vi "New Algo integrated.vi"(0 "Result data in":T6={"Measurement Names Array"=[], "Pass-Fail Array"=[], "Measurement Values Array "=[], "Roi for overlay (Arrows) Array"=[], "Algo Type Array"=[], "Image Array"=[], "Clamp operations"=enum."Average Clamp", "  Search Direction "=[], "Images_Array_in"=[], "ResultPF"=FALSE, "Total Cluster Values"={"Total Fail"=0, "Total Pass"=0, "Total Count"=0}, "Reel Counter Cluster"={"Reel Fail"=0, "Reel Pass"=0, "Reel Count"=0}, "Tolerance  Array"=[], "Array of Cam Spec Control Bool"=[], "Control Pass Fail Array"=[], "Specification Pass Fail Array"=[], "Overlay Arrow Lines"=[], "Camera ID"=[], "Trigger count"=0, "Specification fail?"=FALSE}, 1 "Measurements":T3, 2 "Coordinate Other Cluster":T1, 4 "Calibrated Image":T5[](array[typedef]), 5 "Co Ordinate System":T2(array[cluster]), 7 "error in":errorcluster) -> (21 "Spec Values":T4(array[cluster]), 25 "Result data out":T6={"Measurement Names Array"=[], "Pass-Fail Array"=[], "Measurement Values Array "=[], "Roi for overlay (Arrows) Array"=[], "Algo Type Array"=[], "Image Array"=[], "Clamp operations"=enum."Average Clamp", "  Search Direction "=[], "Images_Array_in"=[], "ResultPF"=FALSE, "Total Cluster Values"={"Total Fail"=0, "Total Pass"=0, "Total Count"=0}, "Reel Counter Cluster"={"Reel Fail"=0, "Reel Pass"=0, "Reel Count"=0}, "Tolerance  Array"=[], "Array of Cam Spec Control Bool"=[], "Control Pass Fail Array"=[], "Specification Pass Fail Array"=[], "Overlay Arrow Lines"=[], "Camera ID"=[], "Trigger count"=0, "Specification fail?"=FALSE}, 27 "error Out":errorcluster)   [LabVIEW 2019, in "Algorithm.lvclass"]
uses:
  FrameworkOverrides/Algorithm.lvclass
  <vilib>/vision/NI_Vision_Development_Module.lvlib
  <vilib>/vision/Image Controls.llb/IMAQ Image.ctl
  Controls/Result Cluster.ctl
  Controls/Measurements JSON Read.ctl
panel:
  out "Numeric":i32
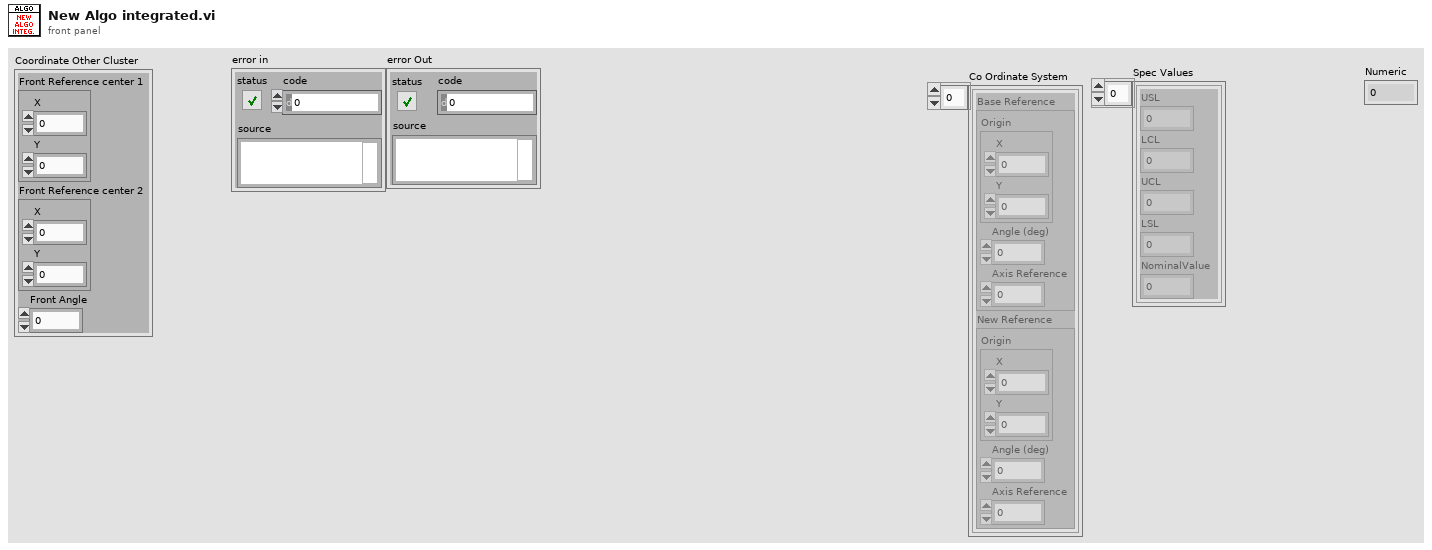
[diagram p1: front panel]
types:
  T1 = cluster{"Front Reference center 1":cluster{"X":sgl, "Y":sgl}, "Front Reference center 2":cluster{"X":sgl, "Y":sgl}, "Front Angle":dbl}
  T2 = cluster{"Base Reference":cluster{"Origin":cluster{"X":sgl, "Y":sgl}, "Angle (deg)":sgl, "Axis Reference":u32}, "New Reference":cluster{"Origin":cluster{"X":sgl, "Y":sgl}, "Angle (deg)":sgl, "Axis Reference":u32}}[]
  T3 = typedef "Algorithm.lvclass/Measurements JSON Read.ctl" = cluster{"RackID":i32, "ImageID":i32, "CameraID":i32, "MeasurementId":i32, "Name":string, "AlgoName":string, "Type":string, "MeasurementEnable":bool, "AlgorithmSequence":cluster{"RefernceEdge":cluster{"Enable":bool, "Method":string, "RefROI":cluster{"Left":i32, "Top":i32, "Right":i32, "Bottom":i32, "Rotation":dbl}, "EdgeOptions":cluster{"EdgePoarity":i32, "KernelSize":i32, "Width":i32, "MinimumEdgeStrength":i32, "InterpolationType":i32, "DataProcessingMethod":i32}, "LineOptions":cluster{"NumberofLines":i32, "Type":i32, "MinScore":i32, "MaxScore":i32, "Orientation":i32, "AngleRange":i32, "AngleTolerance":i32, "StepSize":i32, "MinSNR":i32, "MinPoints":i32, "HoughIterations":i32}, "SearchDirection":i32}, "Measurement":cluster{"ROI1":cluster{"Enable":bool, "ROI":cluster{"Left":i32, "Top":i32, "Right":i32, "Bottom":i32, "Rotation":dbl}, "EdgeOptions":cluster{"EdgePoarity":i32, "KernelSize":i32, "Width":i32, "MinimumEdgeStrength":i32, "InterpolationType":i32, "DataProcessingMethod":i32}, "LineOptions":cluster{"NumberofLines":i32, "Type":i32, "MinScore":i32, "MaxScore":i32, "Orientation":i32, "AngleRange":i32, "AngleTolerance":i32, "StepSize":i32, "MinSNR":i32, "MinPoints":i32, "HoughIterations":i32}, "Process":i32, "StepSize":i32, "SearchDirection":i32, "CircleEdgeOptions":cluster{"SearchDirection":i32, "EdgeOptions":cluster{"EdgePoarity":i32, "KernelSize":i32, "Width":i32, "MinimumEdgeStrength":i32, "InterpolationType":i32, "DataProcessingMethod":i32}}, "CircleFitOptions":cluster{"Process":i32, "StepSize":i32, "MAxPixelRadius":dbl}, "CircleSearchDirection":i32, "CurveParameters":cluster{"ExtractionMode":i32, "EdgeThreshold":i32, "EdgeFilterSize":i32, "MinLength":i32, "RowSearchStepSize":i32, "ColSearchStepSize":i32, "MaxEndpointGap":i32, "Closed":bool, "Subpixel":bool}, "MinimumMatchScore":i32, "CircleDescriptor":cluster{"MinRadius":i32, "MaxRadius":i32}, "EllipseDescriptor":cluster{"MinMajorRadius":i32, "MaxMajorRadius":i32, "MinMinorRadius":i32, "MaxMinorRadius":i32}}, "ROI2":cluster{"Enable":bool, "ROI":cluster{"Left":i32, "Top":i32, "Right":i32, "Bottom":i32, "Rotation":dbl}, "EdgeOptions":cluster{"EdgePoarity":i32, "KernelSize":i32, "Width":i32, "MinimumEdgeStrength":i32, "InterpolationType":i32, "DataProcessingMethod":i32}, "LineOptions":cluster{"NumberofLines":i32, "Type":i32, "MinScore":i32, "MaxScore":i32, "Orientation":i32, "AngleRange":i32, "AngleTolerance":i32, "StepSize":i32, "MinSNR":i32, "MinPoints":i32, "HoughIterations":i32}, "Process":i32, "StepSize":i32, "SearchDirection":i32, "CircleEdgeOptions":cluster{"SearchDirection":i32, "EdgeOptions":cluster{"EdgePoarity":i32, "KernelSize":i32, "Width":i32, "MinimumEdgeStrength":i32, "InterpolationType":i32, "DataProcessingMethod":i32}}, "CircleFitOptions":cluster{"Process":i32, "StepSize":i32, "MAxPixelRadius":dbl}, "CircleSearchDirection":i32, "CurveParameters":cluster{"ExtractionMode":i32, "EdgeThreshold":i32, "EdgeFilterSize":i32, "MinLength":i32, "RowSearchStepSize":i32, "ColSearchStepSize":i32, "MaxEndpointGap":i32, "Closed":bool, "Subpixel":bool}, "MinimumMatchScore":i32, "CircleDescriptor":cluster{"MinRadius":i32, "MaxRadius":i32}, "EllipseDescriptor":cluster{"MinMajorRadius":i32, "MaxMajorRadius":i32, "MinMinorRadius":i32, "MaxMinorRadius":i32}}}}, "MathExpression":cluster{"Algorithm":string, "MathExpression":string, "ResultVariable":string}, "MathCorrectionParameters":cluster{"Radius":dbl, "CurlGap":dbl, "Thickness":dbl, "MeasurementIndices":i32[], "MathAlgoName":string, "MathAlgoFormula":string, "CorrectionForAngle":i32[], "NumericAray":i32[], "StringArray":string[]}, "ResultVariableCluster":cluster{"RVName":string, "RVSequence":string, "RVIndex":i32, "RVID":i32, "RVValue":dbl}, "CalibrationCoefficients":cluster{"A1":dbl, "A2":dbl, "A3":dbl}, "UserCalibCoefficients":cluster{"UserCorrectionLinearityCoeff":dbl, "UserCorrectionBiasCoeff":dbl}, "SpecValues":cluster{"LCL":dbl, "UCL":dbl, "LSL":dbl, "USL":dbl, "NominalValue":dbl}, "OverlayOptions":cluster{"OverlayEnable":bool, "OverlayText":string, "OverlayCoords":i32[], "OverlayAngle":i32, "OverlayTextSize":i32, "OverlayTextColor":string, "OverlayROI":bool, "OverlayRakeLine":bool, "OverlayPoints":bool}, "DatalogEnable":bool, "DisplayIcon":string}[]
  T4 = cluster{"USL":dbl, "LCL":dbl, "UCL":dbl, "LSL":dbl, "NominalValue":dbl}[]
  T5 = typedef "IMAQ Image.ctl" = refnum<image>
  T6 = typedef "Algorithm.lvclass/Result Cluster.ctl" = cluster{"Measurement Names Array":string[], "Pass-Fail Array":bool[], "Measurement Values Array ":dbl[], "Roi for overlay (Arrows) Array":cluster{"Points for Arrow Overlay[0]":cluster{"x":dbl, "y":dbl}, "Points for Arrow Overlay[1]":cluster{"x":dbl, "y":dbl}, "Points for Arrow Overlay[2]":cluster{"x":dbl, "y":dbl}, "Points for Arrow Overlay[3]":cluster{"x":dbl, "y":dbl}}[], "Algo Type Array":string[], "Image Array":string[], "Clamp operations":enum16{"Min Clamp", "Max Clamp", "Average Clamp"}, "  Search Direction ":enum16{"Left to Right", "Right to Left", "Top to Bottom", "Bottom to Top"}[], "Images_Array_in":T5[], "ResultPF":bool, "Total Cluster Values":cluster{"Total Fail":u64, "Total Pass":u64, "Total Count":u64}, "Reel Counter Cluster":cluster{"Reel Fail":u64, "Reel Pass":u64, "Reel Count":u64}, "Tolerance  Array":string[], "Array of Cam Spec Control Bool":cluster{"Specification Boolean":bool, "Control Boolean":bool, "Camera ID":i8}[], "Control Pass Fail Array":bool[], "Specification Pass Fail Array":bool[], "Overlay Arrow Lines":cluster{"First Overlay Line ":cluster{"Start Point":cluster{"X":sgl, "Y":sgl}, "Start Point":cluster{"X":sgl, "Y":sgl}}, "Second Overlay Line ":cluster{"Start Point":cluster{"X":sgl, "Y":sgl}, "Start Point":cluster{"X":sgl, "Y":sgl}}}[], "Camera ID":i8[], "Trigger count":i32, "Specification fail?":bool}
  T7 = typedef "ROI Descriptor" = cluster{"Global Rectangle":i32[], "Contours":cluster{"ID":enum32{"External", "Internal"}, "Type":u32, "Coordinates":i32[]}[]}
  T8 = cluster{"ROI Ref [ After Transformation]":T7, "Measurement ROI 1 [After Transformation]":T7, "Measurement ROI 2 [After Transformation]":T7}
  T9 = typedef "Edge Options.ctl" = cluster{"Edge Polarity":T10, "Kernel Size":u32, "Width":u32, "Minimum Edge Strength":sgl, "Interpolation Type":enum32{"Zero Order", "Bilinear", "Quadratic", "Cubic", "Bilinear Fixed"}, "Data Processing Method":enum32{"Average", "Median"}}
  T10 = typedef "Edge Polarity.ctl" = u32
  T11 = typedef "Straight Edge Options.ctl" = cluster{"Number of Lines":i32, "Type":T12, "Min. Score":dbl, "Max. Score":dbl, "Orientation":dbl, "Angle Range":dbl, "Angle Tolerance":dbl, "Step Size":u32, "Min. SNR (db)":dbl, "Min. Points (%)":dbl, "Hough Iterations":i32}
  T12 = typedef "Straight Edge Process.ctl" = enum32{"First Edge Rake", "Best Edge Rake", "Hough Edge Rake", "First Edge Projection", "Best Edge Projection"}
  T13 = cluster{"RackID":i32, "ImageID":i32, "CameraID":i32, "MeasurementID":i32, "Measurement Name":string, "Algo Name":string, "Algo Type":string, "Ref ROI Cluster":cluster{"ROI Ref":cluster{"Global Rectangle":i32[], "Contours":cluster{"ID":enum32{"External", "Internal"}, "Type":u32, "Coordinates":i32[]}[]}, "Edge Options ROI Ref":T9, "Line Options ROI Ref":T11, "Search Direction ROI Ref":u32, "RefROIEnable":bool}, "Measurement ROI 1 Cluster":cluster{"Meas ROI 1":T7, "Edge Options ROI 1":T9, "Line Options ROI 1":T11, "Scan/Search Direction ROI 1":u16, "Step Size ROI 1":u32, "Process ROI 1":enum16{"Get First Edge", "Get First + Last Edge", "Get All Edges", "Get Best Edge"}, "Circle Options ROI 1":cluster{"Search  Direction":u32, "Edge Options":T9, "Show Search Area":bool, "Show Search Lines":bool, "Show Edges Found":bool, "Show Result":bool, "Search Area Color":u32, "Search Lines Color":u32, "Edge Locations Color":u32, "Result Color":u32, "Overlay Group Name":string}, "Circle Fit Options ROI 1":cluster{"Process":enum16{"Get First Edge", "Get First + Last Edge", "Get All Edges", "Get Best Edge"}, "Step Size":dbl, "Max Pixel Radius":i32}}, "Measurement ROI 2 Cluster":cluster{"Meas ROI 2":T7, "Edge Options ROI 2":T9, "Line Options ROI 2":T11, "Scan/Search Direction ROI 2":u32, "Step Size ROI 2":u32, "Process ROI 2":enum16{"Get First Edge", "Get First + Last Edge", "Get All Edges", "Get Best Edge"}, "Circle Options ROI 2":cluster{"Search  Direction":u32, "Edge Options":T9, "Show Search Area":bool, "Show Search Lines":bool, "Show Edges Found":bool, "Show Result":bool, "Search Area Color":u32, "Search Lines Color":u32, "Edge Locations Color":u32, "Result Color":u32, "Overlay Group Name":string}, "Circle Fit Options ROI 2":cluster{"Process":enum16{"Get First Edge", "Get First + Last Edge", "Get All Edges", "Get Best Edge"}, "Step Size":dbl, "Max Pixel Radius":i32}}, "OverlayOptions":cluster{"OverlayEnable":bool, "OverlayText":string, "OverlayCoords":i32[], "OverlayAngle":i32, "OverlayTextSize":i32, "OverlayTextColor":string, "OverlayROI":bool, "OverlayRakeLine":bool, "OverlayPoints":bool}, "MathExpression":cluster{"Algorithm":string, "MathExpression":string, "ResultVariable":string}, "MathCorrectionParameters":cluster{"Radius":dbl, "CurlGap":dbl, "Thickness":dbl, "MeasurementIndices":i32[], "MathAlgoName":string, "MathAlgoFormula":string, "CorrectionForAngle":i32[], "NumericAray":i32[], "StringArray":string[]}, "ResultVariableCluster":cluster{"RVName":string, "RVSequence":string, "RVIndex":i32, "RVID":i32, "RVValue":dbl}, "CalibrationCoefficients":cluster{"A1":dbl, "A2":dbl, "A3":dbl}, cluster{"UserCalibCoefficients":cluster{"UserCorrectionLinearityCoeff":dbl, "UserCorrectionBiasCoeff":dbl}}, "SpecValues":cluster{"LCL":dbl, "UCL":dbl, "LSL":dbl, "USL":dbl, "NominalValue":dbl}}
  T14 = cluster{"ROI Ref":cluster{"Global Rectangle":i32[], "Contours":cluster{"ID":enum32{"External", "Internal"}, "Type":u32, "Coordinates":i32[]}[]}, "Edge Options ROI Ref":T9, "Line Options ROI Ref":T11, "Search Direction ROI Ref":u32, "RefROIEnable":bool}
  T15 = cluster{"Meas ROI 1":T7, "Edge Options ROI 1":T9, "Line Options ROI 1":T11, "Scan/Search Direction ROI 1":u16, "Step Size ROI 1":u32, "Process ROI 1":enum16{"Get First Edge", "Get First + Last Edge", "Get All Edges", "Get Best Edge"}, "Circle Options ROI 1":cluster{"Search  Direction":u32, "Edge Options":T9, "Show Search Area":bool, "Show Search Lines":bool, "Show Edges Found":bool, "Show Result":bool, "Search Area Color":u32, "Search Lines Color":u32, "Edge Locations Color":u32, "Result Color":u32, "Overlay Group Name":string}, "Circle Fit Options ROI 1":cluster{"Process":enum16{"Get First Edge", "Get First + Last Edge", "Get All Edges", "Get Best Edge"}, "Step Size":dbl, "Max Pixel Radius":i32}}
  T16 = cluster{"Meas ROI 2":T7, "Edge Options ROI 2":T9, "Line Options ROI 2":T11, "Scan/Search Direction ROI 2":u32, "Step Size ROI 2":u32, "Process ROI 2":enum16{"Get First Edge", "Get First + Last Edge", "Get All Edges", "Get Best Edge"}, "Circle Options ROI 2":cluster{"Search  Direction":u32, "Edge Options":T9, "Show Search Area":bool, "Show Search Lines":bool, "Show Edges Found":bool, "Show Result":bool, "Search Area Color":u32, "Search Lines Color":u32, "Edge Locations Color":u32, "Result Color":u32, "Overlay Group Name":string}, "Circle Fit Options ROI 2":cluster{"Process":enum16{"Get First Edge", "Get First + Last Edge", "Get All Edges", "Get Best Edge"}, "Step Size":dbl, "Max Pixel Radius":i32}}
  T17 = cluster{"Base Reference":cluster{"Origin":cluster{"X":sgl, "Y":sgl}, "Angle (deg)":sgl, "Axis Reference":u32}, "New Reference":cluster{"Origin":cluster{"X":sgl, "Y":sgl}, "Angle (deg)":sgl, "Axis Reference":u32}}
  T18 = cluster{"Global Rectangle":i32[], "Contours":cluster{"ID":enum32{"External", "Internal"}, "Type":u32, "Coordinates":i32[]}[]}
  T19 = cluster{"Origin":cluster{"X":sgl, "Y":sgl}, "Angle (deg)":sgl, "Axis Reference":u32}
  T20 = cluster{"Point1 (Pixels)":cluster{"X":sgl, "Y":sgl}, "Point2 (Pixels)":cluster{"X":sgl, "Y":sgl}, "Point1 (Real-World)":cluster{"X":sgl, "Y":sgl}, "Point2 (Real-World)":cluster{"X":sgl, "Y":sgl}, "Angle (Pixel)":dbl, "Angle (Real-World)":dbl, "Score":dbl, "Straightness":dbl, "Average SNR (db)":dbl, "Calibration Valid":bool}[]
  T21 = cluster{"Point1 (Pixels)":cluster{"X":sgl, "Y":sgl}, "Point2 (Pixels)":cluster{"X":sgl, "Y":sgl}, "Point1 (Real-World)":cluster{"X":sgl, "Y":sgl}, "Point2 (Real-World)":cluster{"X":sgl, "Y":sgl}, "Angle (Pixel)":dbl, "Angle (Real-World)":dbl, "Score":dbl, "Straightness":dbl, "Average SNR (db)":dbl, "Calibration Valid":bool}
  T22 = typedef "IMAQ Rectangle" = cluster{"Left":i32, "Top":i32, "Right":i32, "Bottom":i32, "Rotation":dbl}
  T23 = cluster{"First Overlay Line ":cluster{"Start Point":cluster{"X":sgl, "Y":sgl}, "Start Point":cluster{"X":sgl, "Y":sgl}}, "Second Overlay Line ":cluster{"Start Point":cluster{"X":sgl, "Y":sgl}, "Start Point":cluster{"X":sgl, "Y":sgl}}}
  T24 = cluster{"LCL":dbl, "UCL":dbl, "LSL":dbl, "USL":dbl, "NominalValue":dbl}
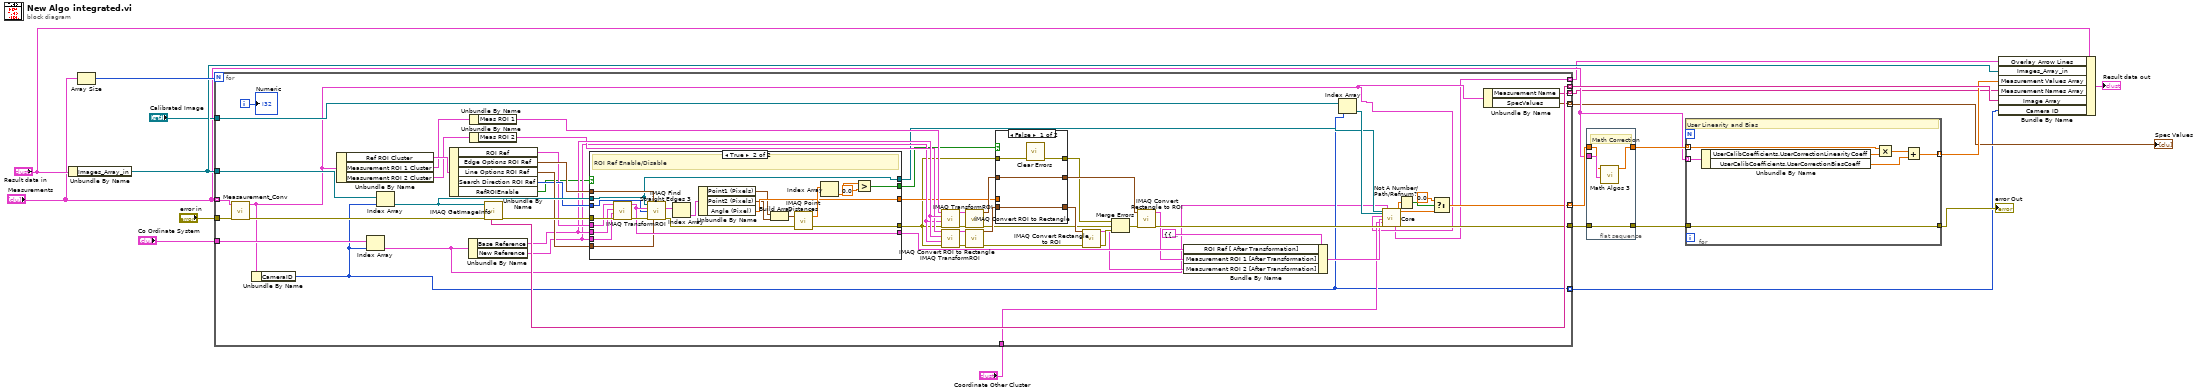
[diagram p0: block diagram]
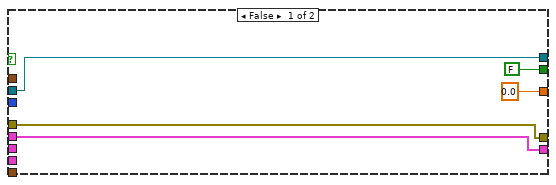
[diagram p2: hidden frame]
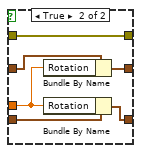
[diagram p3: hidden frame]
diagram:
  n1 = Unbundle By Name("Result data in") -> ("Images_Array_in"=w14:T5[])
  n2 = Array Size(array="Measurements") -> (size(s)=w15:i32)
  n3 = for {
    N: w15 -> [_]
    tunnel: w14 -> [w78]
    tunnel: "error in" -> [w69]
    tunnel: [w74] -> w10
    tunnel: [w75] -> w18 mode=indexing
    tunnel: "Calibrated Image" -> [w77]
    tunnel: [w73] -> w11 mode=indexing
    tunnel: "Measurements" -> [w68] mode=indexing
    tunnel: "Co Ordinate System" -> [w66]
    tunnel: [w50] -> w5 mode=indexing
    tunnel: [w49] -> w6 mode=indexing
    tunnel: "Coordinate Other Cluster" -> [w48]
    tunnel: [w23] -> w2 mode=indexing
    tunnel: [w22] -> w1 mode=indexing
    i -> [w76]
    n4 = call "Measaurement_Conv.vi"("error in (no error)"=w69, "Measurements"=w68) -> ("error in (no error)"=w67:errorcluster, "Measurement JSON Data"=w47:T13)  [unwired: 8 in]
    n5 = Unbundle By Name(w47) -> ("CameraID"=w22:i32)
    n6 = Unbundle By Name(w47) -> ("Ref ROI Cluster"=w54:T14, "Measurement ROI 1 Cluster"=w53:T15, "Measurement ROI 2 Cluster"=w52:T16)
    n7 = Index Array(array=w66, index=w22) -> (element=w21:T17)
    n8 = Index Array(array=w78, index=w22) -> (element=w70:T5)
    n9 = Unbundle By Name(w54) -> ("ROI Ref"=w61:T18, "Edge Options ROI Ref"=w64:T9, "Line Options ROI Ref"=w63:T11, "Search Direction ROI Ref"=w62:u32, "RefROIEnable"=w55:bool)
    n10 = Unbundle By Name(w21) -> ("Base Reference"=w60:T19, "New Reference"=w57:T19)
    n11 = Unbundle By Name(w53) -> ("Meas ROI 1"=w59:T7)
    n12 = Unbundle By Name(w52) -> ("Meas ROI 2"=w58:T7)
    n13 = call "IMAQ GetImageInfo"("error in (no error)"=w67, "Image"=w70) -> ("error out"=w72:errorcluster, "Image Name"=w75:string)  [unwired: 2 in, 6 out]
    n14 = case shown="True" w55 {
      tunnel: [FALSE w105] -> w40
      tunnel: [0.0 ("Angle (Pixel)") w97] -> w32
      tunnel: [w83 w96] -> w31
      tunnel: [w80 w95] -> w27
      tunnel: w72 -> [w80 w91]
      tunnel: w63 -> [_ w90]
      tunnel: w62 -> [_ w89]
      tunnel: w64 -> [_ w88]
      tunnel: w61 -> [w83 w87]
      tunnel: w60 -> [_ w86]
      tunnel: w57 -> [_ w85]
      tunnel: w70 -> [w79 w84]
      tunnel: [w79 w84] -> w56
      frame False {
      }
      frame True {
        # "ROI Ref Enable/Disable"
        n15 = call "IMAQ TransformROI"("error in (no error)"=w91, "New Reference"=w85, "Base Reference"=w86, "ROI Descriptor"=w87) -> ("error out"=w100:errorcluster, "ROI Descriptor out"=w96:T7)  [unwired: 6 in]
        n16 = call "IMAQ Find Straight Edges 3"("Image"=w84, "Edge Options"=w88, "ROI Descriptor"=w96, "Search Direction"=w89, "error in (no error)"=w100, "Line Options"=w90) -> ("Straight Edges"=w99:T20, "error out"=w101:errorcluster)  [unwired: 5 in, 3 out]
        n17 = Index Array(array=w99) -> (element=w98:T21)  [unwired: 1 in]
        n18 = Unbundle By Name(w98) -> ("Point1 (Pixels)"=w94:cluster{"X":sgl, "Y":sgl}, "Point2 (Pixels)"=w93:cluster{"X":sgl, "Y":sgl}, "Angle (Pixel)"=w97:dbl)
        n19 = Build Array(w94, w93) -> (w92:cluster{"X":sgl, "Y":sgl}[])
        n20 = call "IMAQ Point Distances"("Points"=w92, "error in (no error)"=w101) -> ("Distances"=w104:sgl[], "error out"=w95:errorcluster)  [unwired: 3 in]
        n21 = Index Array(array=w104) -> (element=w103:sgl)  [unwired: 1 in]
        n22 = Greater?(x=w103, y=sgl 0.0) -> (0:w105:bool)
      }
    }
    n23 = call "IMAQ TransformROI"("error in (no error)"=w27, "New Reference"=w57, "Base Reference"=w60, "ROI Descriptor"=w59) -> ("error out"=w46:errorcluster, "ROI Descriptor out"=w42:T7)  [unwired: 6 in]
    n24 = call "IMAQ TransformROI"("error in (no error)"=w27, "New Reference"=w57, "Base Reference"=w60, "ROI Descriptor"=w58) -> ("error out"=w44:errorcluster, "ROI Descriptor out"=w45:T7)  [unwired: 6 in]
    n25 = call "IMAQ Convert ROI to Rectangle"("error in (no error)"=w46, "ROI Descriptor"=w42) -> ("error out"=w34:errorcluster, "Rectangle"=w38:T22)  [unwired: 7 in]
    n26 = call "IMAQ Convert ROI to Rectangle"("error in (no error)"=w44, "ROI Descriptor"=w45) -> ("error out"=w43:errorcluster, "Rectangle"=w39:T22)  [unwired: 7 in]
    n27 = case shown="False" w40 {
      tunnel: w39 -> [w109 w115]
      tunnel: w38 -> [w108 w114]
      tunnel: [w109 w113] -> w37
      tunnel: [w108 w112] -> w36
      tunnel: w27 -> [w107 w110]
      tunnel: [w106 w110] -> w35
      tunnel: w32 -> [_ w111]
      frame False {
        n28 = call <vilib>:"Clear Errors.vi"("error in (no error)"=w107) -> ("error out"=w106:errorcluster)  [unwired: 5 in, 1 out]
      }
      frame True {
        n29 = Bundle By Name(cluster=w114, "Rotation"=w111) -> (w112:T22)
        n30 = Bundle By Name(cluster=w115, "Rotation"=w111) -> (w113:T22)
      }
    }
    n31 = call "IMAQ Convert Rectangle to ROI"("error in (no error)"=w43, "Rectangle"=w37) -> ("error out"=w33:errorcluster, "ROI Descriptor"=w29:T7)  [unwired: 7 in]
    n32 = Merge Errors(w35, w34, w33) -> (w41:errorcluster)
    n33 = call "IMAQ Convert Rectangle to ROI"("error in (no error)"=w41, "Rectangle"=w36) -> ("error out"=w65:errorcluster, "ROI Descriptor"=w30:T7)  [unwired: 7 in]
    n34 = Bundle By Name(cluster=T8 {"ROI Ref [ After Transformation]"={"Global Rectangle"=[], "Contours"=[]}, "Measurement ROI 1 [After Transformation]"={"Global Rectangle"=[], "Contours"=[]}, "Measurement ROI 2 [After Transformation]"={"Global Rectangle"=[], "Contours"=[]}}, "ROI Ref [ After Transformation]"=w31, "Measurement ROI 1 [After Transformation]"=w30, "Measurement ROI 2 [After Transformation]"=w29) -> (w51:T8)
    n35 = Index Array(array=w77, index=w22) -> (element=w71:T5)
    n36 = call "Core.vi"("Image In"=w56, "CalibratedImage In"=w71, "Measurement JSON Data"=w47, "Transformed ROI cluster"=w51, "Coordinate Other Cluster"=w48, "error in (no error)"=w65, "coordinate system"=w21) -> ("Overlay Arrow Lines"=w23:T23, "Numeric"=w24:sgl, "error out"=w74:errorcluster)  [unwired: 10 in]
    n37 = Not A Number/Path/Refnum?(number/path/refnum=w24) -> (NaN/Path/Refnum?=w26:bool)
    n38 = Select(t=sgl 0.0, s=w26, f=w24) -> (s? t:f=w73:sgl)
    n39 = Unbundle By Name(w47) -> ("Measurement Name"=w49:string, "SpecValues"=w50:T24)
    "Numeric" <- w76
  }
  "Spec Values" <- w5
  n40 = flat-sequence {
    tunnel: [w119] -> w12
    tunnel: "Measurements" -> [w118]
    tunnel: w11 -> [w117]
    tunnel: w10 -> [w116]
    tunnel: [w116] -> w9
    frame #0 {
      # "Math Correction"
      n41 = call "Math Algos 3.vi"("Measurements 2"=w118, "W (from Top View Algo)"=w117) -> ("H corrected"=w119:dbl[])  [unwired: 9 in]
    }
  }
  n42 = for {
    tunnel: "Measurements" -> [w126] mode=indexing
    tunnel: w12 -> [w125] mode=indexing
    tunnel: [w121] -> w16 mode=indexing
    tunnel: w9 -> [w120]
    tunnel: [w120] -> w3
    # "User Linearity and Bias"
    n43 = Unbundle By Name(w126) -> ("UserCalibCoefficients.UserCorrectionLinearityCoeff"=w124:dbl, "UserCalibCoefficients.UserCorrectionBiasCoeff"=w122:dbl)
    n44 = Multiply(x=w125, y=w124) -> (x*y=w123:dbl)
    n45 = Add(x=w123, y=w122) -> (x+y=w121:dbl)
  }
  "error Out" <- w3
  n46 = Bundle By Name(cluster="Result data in", "Overlay Arrow Lines"=w2, "Images_Array_in"=w14, "Measurement Values Array"=w16, "Measurement Names Array"=w6, "Image Array"=w18, "Camera ID"=w1) -> (→"Result data out":T6)
